vi "Begin.vi"() -> (0 "error out":errorcluster)   [LabVIEW 2013]
doc: "Called before other user functions, this VI is expected to open initial I/O refnums, load in file data, and do all program initialization. Notice that the <B>error out</B> terminal is simply used for data flow. Wiring it to other structures or subVIs ensures that this VI runs first."
uses:
  <vilib>/Rock Robotics/WPI/DriverStation/WPI_DriverStationRobotMode2.ctl
  <vilib>/Rock Robotics/WPI/Joystick/WPI_JoystickDeviceEnum.ctl
  <vilib>/Rock Robotics/SystemInterfaces/AI/FPGA_AIGyroChannel.ctl
  <vilib>/Rock Robotics/SystemInterfaces/Typedef/FPGA_TypedefAnalogModuleForGyro.ctl
  <vilib>/Rock Robotics/SystemInterfaces/DIO/FPGA_DIOChannel.ctl
  <vilib>/Rock Robotics/SystemInterfaces/DIO/FPGA_DIORelayChannel.ctl
  <vilib>/Rock Robotics/SystemInterfaces/AI/FPGA_AIChannel.ctl
  <vilib>/Rock Robotics/SystemInterfaces/DIO/FPGA_DIOPWMChannel.ctl
  <vilib>/Rock Robotics/SystemInterfaces/Typedef/FPGA_TypedefDigitalModule.ctl
  Drivetrain/Arcade Drive Ref.ctl
  <vilib>/Rock Robotics/WPI/MotorControl/WPI_MotorControlDeviceRef.ctl
  <vilib>/Rock Robotics/WPI/PWM/WPI_PWMDeadband.ctl
  <vilib>/Rock Robotics/WPI/CAN/Jaguar/SubVIs/WPI_CANJaguar_ControlMode.ctl
  <vilib>/Rock Robotics/WPI/PWM/WPI_PWMTransform_ConPane.ctl
  <vilib>/Rock Robotics/WPI/Solenoid/WPI_SolenoidChannel.ctl
  Robot Global Data.vi
  <vilib>/Rock Robotics/WPI/MotorControl/WPI_MotorControlOpen Talon.vi
  <vilib>/Rock Robotics/WPI/Counter/WPI_CounterDigitalInputToDigitalSource.vi
  <vilib>/Rock Robotics/WPI/Solenoid/WPI_SolenoidOpenSingle.vi
  <vilib>/Rock Robotics/WPI/Compressor/WPI_CompressorGetSetRefNum.vi
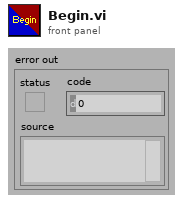
[diagram p1: front panel]
types:
  T1 = typedef "WPI_SolenoidChannel.ctl" = enum8{"Solenoid 1", "Solenoid 2", "Solenoid 3", "Solenoid 4", "Solenoid 5", "Solenoid 6", "Solenoid 7", "Solenoid 8", "Invalid"}
  T2 = typedef "Arcade Drive Ref.ctl" = cluster{"L1":T3, "L2":T3, "R1":T3, "R2":T3, "Motor Count":enum16{"2 Motor", "4 Motor"}, "L Reversed?":bool, "R Reversed?":bool}
  T3 = typedef "WPI_MotorControlDeviceRef.ctl" = cluster{"DeviceStatus":errorcluster, "Type":enum16{"PWM", "CAN"}, "PWM":cluster{"Digital Module":T4, "PWM Channel":T5, "DeadBand":T6}, "CAN":cluster{"Device Number":u8, "Control Mode":T7, "Semaphore":T8, "Max Vout":dbl}, "Invert":bool, "TransformRef":T9, "InvTransformRef":T9}
  T4 = typedef "FPGA_TypedefDigitalModule.ctl" = enum16{"Digital Module 1", "Digital Module 2"}
  T5 = typedef "FPGA_DIOPWMChannel.ctl" = enum8{"PWM 1", "PWM 2", "PWM 3", "PWM 4", "PWM 5", "PWM 6", "PWM 7", "PWM 8", "PWM 9", "PWM 10", "Invalid"}
  T6 = typedef "WPI_PWMDeadband.ctl" = cluster{"Name":string, "maxPositivePwm":i32, "minPositivePwm":i32, "centerPwm":i32, "maxNegativePwm":i32, "minNegativePwm":i32, "angularRange":u16}
  T7 = typedef "WPI_CANJaguar_ControlMode.ctl" = enum8{"Percent VBus", "Current", "Speed", "Position", "Voltage"}
  T8 = typedef "Semaphore RefNum" = refnum<k1>
  T9 = typedef "WPI_PWMTransform_ConPane.ctl" = refnum<vi>
  T10 = typedef "FPGA_DIOChannel.ctl" = enum8{"DIO 1", "DIO 2", "DIO 3", "DIO 4", "DIO 5", "DIO 6", "DIO 7", "DIO 8", "DIO 9", "DIO 10", "DIO 11", "DIO 12", "DIO 13", "DIO 14", "Invalid"}
  T11 = typedef "FPGA_AIChannel.ctl" = enum8{"AI 1", "AI 2", "AI 3", "AI 4", "AI 5", "AI 6", "AI 7", "AI 8", "Invalid"}
  T12 = typedef "FPGA_DIORelayChannel.ctl" = enum8{"Relay 1", "Relay 2", "Relay 3", "Relay 4", "Relay 5", "Relay 6", "Relay 7", "Relay 8", "Invalid"}
  T13 = typedef "WPI_JoystickDeviceEnum.ctl" = enum16{"USB 1", "USB 2", "USB 3", "USB 4", "Kinect 1", "Kinect 2"}
  T14 = typedef "FPGA_TypedefAnalogModuleForGyro.ctl" = enum16{"Analog Module 1"}
  T15 = typedef "FPGA_AIGyroChannel.ctl" = enum8{"AI 1", "AI 2", "Invalid"}
  T16 = typedef "WPI_DriverStationRobotMode2.ctl" = enum16{"Autonomous Disabled", "Autonomous Enabled", "Teleop Disabled", "Teleop Enabled", "Timeout", "Finish", "Test Disabled", "Test Enabled"}
  T17 = typedef "WPI_DigitalInputDevRef.ctl" = cluster{"DevStatus":errorcluster, "DIO Channel":T10, "Digital Module":T4}
  T18 = typedef "FPGA_CounterEncoderSourceConvertionLVSourceType.ctl" = cluster{"DevStatus":errorcluster, "AnalogTriggerMode?":bool, "DigitalMode":cluster{"Digital Module":T4, "DIO Channel":T19}, "AnalogTriggerMode":cluster{"AnalogTriggerIndex":T20, "OutputType":T21}}
  T19 = typedef "FPGA_DIODigitalSourceChannel.ctl" = enum8{"DIO 1", "DIO 2", "DIO 3", "DIO 4", "DIO 5", "DIO 6", "DIO 7", "DIO 8", "DIO 9", "DIO 10", "DIO 11", "DIO 12", "DIO 13", "DIO 14", "Disabled"}
  T20 = typedef "FPGA_AnalogTriggerIndex.ctl" = enum8{"Trig 0", "Trig 1", "Trig 2", "Trig 3", "Trig 4", "Trig 5", "Trig 6", "Trig 7", "Invalid"}
  T21 = typedef "FPGA_AnalogTriggerOutType.ctl" = enum16{"InWindow", "TriggerState", "Rising", "Falling"}
  T22 = typedef "WPI_EncoderDevRef.ctl" = cluster{"DevStatus":errorcluster, "EncoderIndex":T23, "CounterIndex":T24, "DistancePerCount":dbl, "Decoding Type":T25}
  T23 = typedef "FPGA_EncoderIdx.ctl" = enum8{"Enc 0", "Enc 1", "Enc 2", "Enc 3", "Invalid"}
  T24 = typedef "FPGA_CounterCtrSystemIndex.ctl" = enum8{"Ctr 0", "Ctr 1", "Ctr 2", "Ctr 3", "Ctr 4", "Ctr 5", "Ctr 6", "Ctr 7", "Invalid"}
  T25 = typedef "WPI_EncoderType.ctl" = enum16{"1x", "2x", "4x"}
  T26 = typedef "WPI_AnalogChannelDevRef.ctl" = cluster{"DevStatus":errorcluster, "Analog Module":T27, "Analog Channel":T11}
  T27 = typedef "FPGA_TypedefAnalogModule.ctl" = enum16{"Analog Module 1", "Analog Module 2"}
  T28 = typedef "WPI_JoystickDevRef.ctl" = cluster{"Device":T13}
  T29 = typedef "WPI_I2CDevRef.ctl" = cluster{"DevStatus":errorcluster, "Digital Module":T4, "Device Address":u8}
  T30 = typedef "WPI_SolenoidDevRef.ctl" = cluster{"DevStatus":errorcluster, "Solenoid Module":T31, "Forward Solenoid Channel":T1, "Reverse Solenoid Channel":T1}
  T31 = typedef "FPGA_TypedefSolenoidModule.ctl" = enum16{"Solenoid Module 1", "Solenoid Module 2"}
  T32 = typedef "WPI_GyroDevRef.ctl" = cluster{"DevStatus":errorcluster, "Analog Module":T27, "Analog Channel":T11, "Offset":dbl, "Gain (VoltsPerDegree/Second)":dbl}
  T33 = typedef "WPI_CompressorDevRef.ctl" = cluster{"DevStatus":errorcluster, "DigitalInputDevRef":T17, "RelayDevRef":T34}
  T34 = typedef "WPI_RelayDevRef.ctl" = cluster{"DevStatus":errorcluster, "Relay Channel":T12, "Digital Module":T4, "Relay Direction":T35}
  T35 = typedef "WPI_RelayDirection.ctl" = enum16{"Both directions", "Forward only", "Reverse only"}
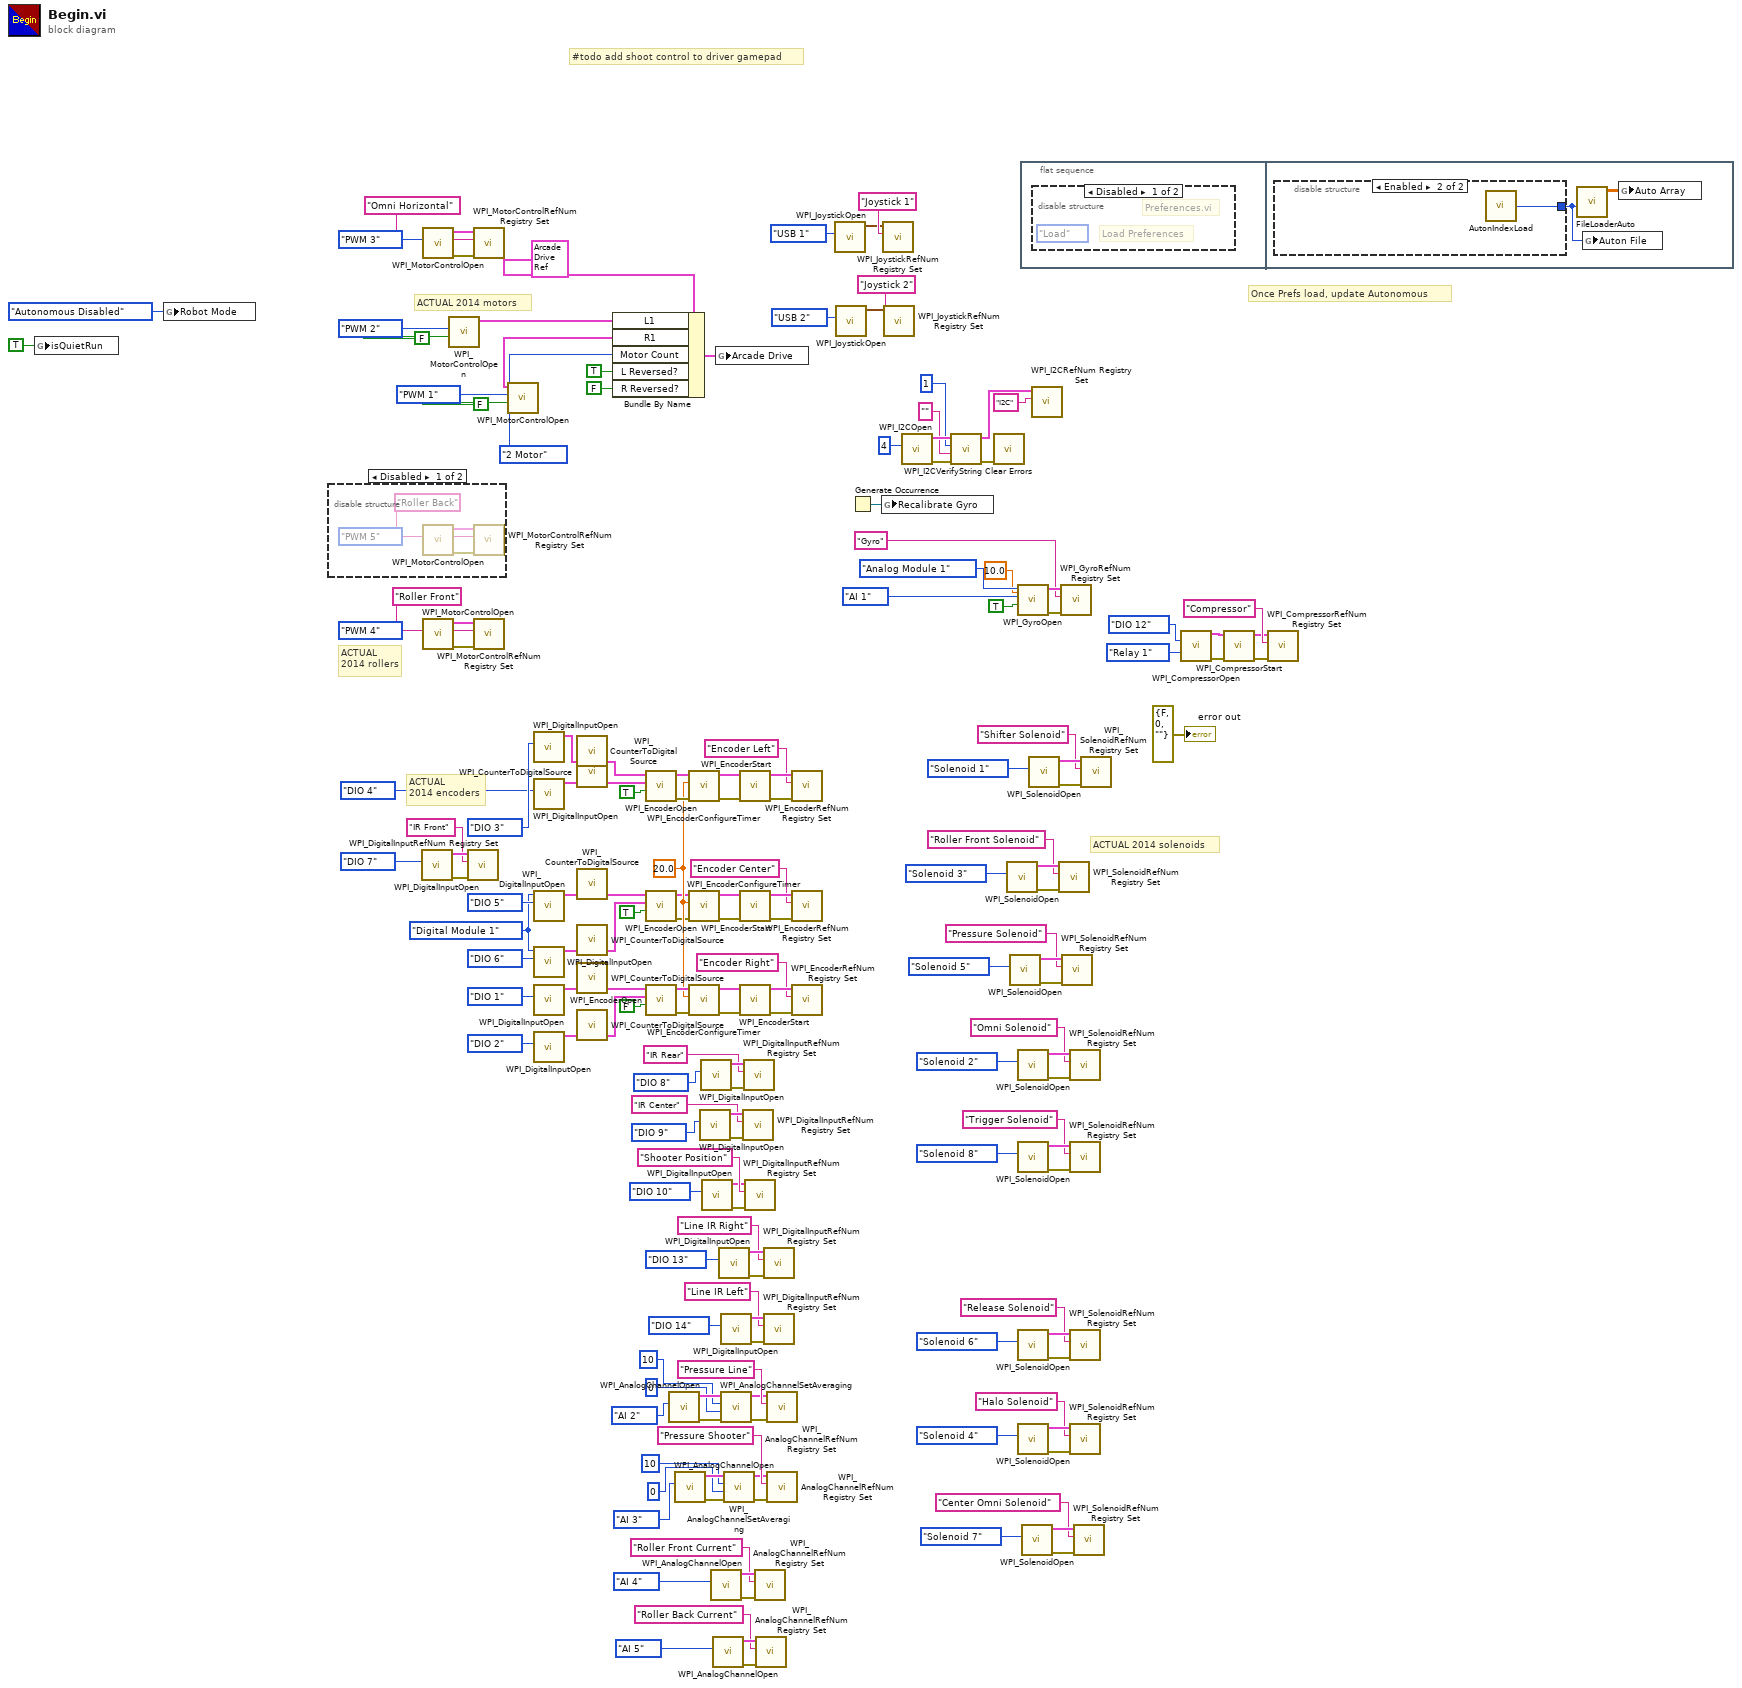
[diagram p0: block diagram]
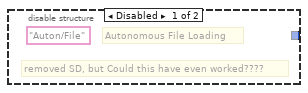
[diagram p4: hidden frame]
diagram:
  w45 = FPGA_TypedefDigitalModule."Digital Module 1" ("Digital Module (Module 1)")
  w95 = 20.0 ("Minimum Rate")
  # "ACTUAL 2014 solenoids"
  # "#todo add shoot control to driver gamepad"
  # "ACTUAL\n2014 encoders"
  # "ACTUAL\n2014 rollers"
  # "ACTUAL 2014 motors"
  # "Once Prefs load, update Autonomous"
  n1 = global write "Robot Global Data.vi" "isQuietRun"(TRUE ("isQuietRun")) -> ()
  n2 = global write "Robot Global Data.vi" "Robot Mode"(WPI_DriverStationRobotMode2."Autonomous Disabled" ("Robot Mode")) -> ()
  n3 = disable-structure shown="Disabled" {
    frame Disabled {
      n4 = call-poly <vilib>:"WPI_MotorControlOpen.vi"("PWM Channel"=FPGA_DIOPWMChannel."PWM 5") -> ("error out"=w179:errorcluster, "MotorControlDeviceRef"=w178:T3)  [unwired: 9 in]
      n5 = call <vilib>:"WPI_MotorControlRefNum Registry Set.vi"("error in (no error)"=w179, "refnum name"="Roller Back", "MotorControlDevRef"=w178) -> ()  [unwired: 7 in, 2 out]
    }
    frame Enabled {
    }
  }
  n6 = call <vilib>:"WPI_DigitalInputOpen.vi"("DIO Channel"=FPGA_DIOChannel."DIO 7") -> ("error out"=w126:errorcluster, "DigitalInputDevRef"=w125:T17)  [unwired: 9 in]
  n7 = call-poly <vilib>:"WPI_MotorControlOpen.vi"("PWM Channel"=FPGA_DIOPWMChannel."PWM 3") -> ("error out"=w49:errorcluster, "MotorControlDeviceRef"=w50:T3)  [unwired: 9 in]
  n8 = call-poly <vilib>:"WPI_MotorControlOpen.vi"("PWM Channel"=FPGA_DIOPWMChannel."PWM 4") -> ("error out"=w132:errorcluster, "MotorControlDeviceRef"=w131:T3)  [unwired: 9 in]
  n9 = call-poly <vilib>:"WPI_MotorControlOpen.vi"("Eliminate Deadband"=FALSE, "PWM Channel"=FPGA_DIOPWMChannel."PWM 2") -> ("MotorControlDeviceRef"=w53:T3)  [unwired: 8 in, 1 out]
  n10 = call <vilib>:"WPI_DigitalInputRefNum Registry Set.vi"("error in (no error)"=w126, "refnum name"="IR Front", "DigitalInputDevRef"=w125) -> ()  [unwired: 7 in, 2 out]
  n11 = call <vilib>:"WPI_MotorControlRefNum Registry Set.vi"("error in (no error)"=w49, "refnum name"="Omni Horizontal", "MotorControlDevRef"=w50) -> ()  [unwired: 7 in, 2 out]
  n12 = call <vilib>:"WPI_MotorControlRefNum Registry Set.vi"("error in (no error)"=w132, "refnum name"="Roller Front", "MotorControlDevRef"=w131) -> ()  [unwired: 7 in, 2 out]
  n13 = call-poly <vilib>:"WPI_MotorControlOpen.vi"("Eliminate Deadband"=FALSE, "PWM Channel"=FPGA_DIOPWMChannel."PWM 1") -> ("MotorControlDeviceRef"=w54:T3)  [unwired: 8 in, 1 out]
  n14 = call <vilib>:"WPI_DigitalInputOpen.vi"("DIO Channel"=FPGA_DIOChannel."DIO 3") -> ("DigitalInputDevRef"=w157:T17)  [unwired: 9 in, 1 out]
  n15 = call <vilib>:"WPI_DigitalInputOpen.vi"("DIO Channel"=FPGA_DIOChannel."DIO 4") -> ("DigitalInputDevRef"=w156:T17)  [unwired: 9 in, 1 out]
  n16 = call <vilib>:"WPI_DigitalInputOpen.vi"("DIO Channel"=FPGA_DIOChannel."DIO 5", "Digital Module (Module 1)"=w45) -> ("DigitalInputDevRef"=w46:T17)  [unwired: 8 in, 1 out]
  n17 = call <vilib>:"WPI_DigitalInputOpen.vi"("DIO Channel"=FPGA_DIOChannel."DIO 6", "Digital Module (Module 1)"=w45) -> ("DigitalInputDevRef"=w43:T17)  [unwired: 8 in, 1 out]
  n18 = call <vilib>:"WPI_DigitalInputOpen.vi"("DIO Channel"=FPGA_DIOChannel."DIO 1") -> ("DigitalInputDevRef"=w164:T17)  [unwired: 9 in, 1 out]
  n19 = call <vilib>:"WPI_DigitalInputOpen.vi"("DIO Channel"=FPGA_DIOChannel."DIO 2") -> ("DigitalInputDevRef"=w165:T17)  [unwired: 9 in, 1 out]
  n20 = call-poly <vilib>:"WPI_CounterToDigitalSource.vi"("DigitalInputDevRef"=w157) -> ("Digital Source"=w158:T18)  [unwired: 6 in]
  n21 = call-poly <vilib>:"WPI_CounterToDigitalSource.vi"("DigitalInputDevRef"=w156) -> ("Digital Source"=w155:T18)  [unwired: 6 in]
  n22 = call-poly <vilib>:"WPI_CounterToDigitalSource.vi"("DigitalInputDevRef"=w46) -> ("Digital Source"=w48:T18)  [unwired: 6 in]
  n23 = call-poly <vilib>:"WPI_CounterToDigitalSource.vi"("DigitalInputDevRef"=w43) -> ("Digital Source"=w42:T18)  [unwired: 6 in]
  n24 = call-poly <vilib>:"WPI_CounterToDigitalSource.vi"("DigitalInputDevRef"=w164) -> ("Digital Source"=w163:T18)  [unwired: 6 in]
  n25 = call-poly <vilib>:"WPI_CounterToDigitalSource.vi"("DigitalInputDevRef"=w165) -> ("Digital Source"=w166:T18)  [unwired: 6 in]
  n26 = Bundle By Name(cluster=T2 {"L1"={"DeviceStatus"={"status"=FALSE, "code"=0, "source"=""}, "Type"=enum."PWM", "PWM"={"Digital Module"=enum."Digital Module 1", "PWM Channel"=enum."PWM 1", "DeadBand"={"Name"="", "maxPositivePwm"=0, "minPositivePwm"=0, "centerPwm"=0, "maxNegativePwm"=0, "minNegativePwm"=0, "angularRange"=0}}, "CAN"={"Device Number"=0, "Control Mode"=enum."Percent VBus", "Semaphore"=refnum, "Max Vout"=0.0}, "Invert"=FALSE, "TransformRef"=refnum, "InvTransformRef"=refnum}, "L2"={"DeviceStatus"={"status"=FALSE, "code"=0, "source"=""}, "Type"=enum."PWM", "PWM"={"Digital Module"=enum."Digital Module 1", "PWM Channel"=enum."PWM 1", "DeadBand"={"Name"="", "maxPositivePwm"=0, "minPositivePwm"=0, "centerPwm"=0, "maxNegativePwm"=0, "minNegativePwm"=0, "angularRange"=0}}, "CAN"={"Device Number"=0, "Control Mode"=enum."Percent VBus", "Semaphore"=refnum, "Max Vout"=0.0}, "Invert"=FALSE, "TransformRef"=refnum, "InvTransformRef"=refnum}, "R1"={"DeviceStatus"={"status"=FALSE, "code"=0, "source"=""}, "Type"=enum."PWM", "PWM"={"Digital Module"=enum."Digital Module 1", "PWM Channel"=enum."PWM 1", "DeadBand"={"Name"="", "maxPositivePwm"=0, "minPositivePwm"=0, "centerPwm"=0, "maxNegativePwm"=0, "minNegativePwm"=0, "angularRange"=0}}, "CAN"={"Device Number"=0, "Control Mode"=enum."Percent VBus", "Semaphore"=refnum, "Max Vout"=0.0}, "Invert"=FALSE, "TransformRef"=refnum, "InvTransformRef"=refnum}, "R2"={"DeviceStatus"={"status"=FALSE, "code"=0, "source"=""}, "Type"=enum."PWM", "PWM"={"Digital Module"=enum."Digital Module 1", "PWM Channel"=enum."PWM 1", "DeadBand"={"Name"="", "maxPositivePwm"=0, "minPositivePwm"=0, "centerPwm"=0, "maxNegativePwm"=0, "minNegativePwm"=0, "angularRange"=0}}, "CAN"={"Device Number"=0, "Control Mode"=enum."Percent VBus", "Semaphore"=refnum, "Max Vout"=0.0}, "Invert"=FALSE, "TransformRef"=refnum, "InvTransformRef"=refnum}, "Motor Count"=enum."2 Motor", "L Reversed?"=FALSE, "R Reversed?"=FALSE} ("Arcade Drive"), "L1"=w53, "R1"=w54, "Motor Count"=enum16{"2 Motor", "4 Motor", ""}."2 Motor", "L Reversed?"=TRUE, "R Reversed?"=FALSE) -> (w73:T2)
  n27 = call <vilib>:"WPI_EncoderOpen.vi"("Invert Direction (False)"=TRUE, "BSource"=w155, "ASource"=w158) -> ("error out"=w160:errorcluster, "EncoderDevRef"=w159:T22)  [unwired: 7 in]
  n28 = call <vilib>:"WPI_EncoderOpen.vi"("Invert Direction (False)"=TRUE, "BSource"=w42, "ASource"=w48) -> ("error out"=w40:errorcluster, "EncoderDevRef"=w41:T22)  [unwired: 7 in]
  n29 = call <vilib>:"WPI_EncoderOpen.vi"("Invert Direction (False)"=FALSE, "BSource"=w166, "ASource"=w163) -> ("error out"=w168:errorcluster, "EncoderDevRef"=w167:T22)  [unwired: 7 in]
  n30 = call <vilib>:"WPI_AnalogChannelOpen.vi"("Analog Channel"=FPGA_AIChannel."AI 2") -> ("error out"=w84:errorcluster, "AIDeviceRef"=w83:T26)  [unwired: 9 in]
  n31 = call <vilib>:"WPI_AnalogChannelOpen.vi"("Analog Channel"=FPGA_AIChannel."AI 3") -> ("error out"=w79:errorcluster, "AIDeviceRef"=w78:T26)  [unwired: 9 in]
  n32 = call <vilib>:"WPI_EncoderConfigureTimer.vi"("error in (no error)"=w160, "Minimum Rate"=w95, "EncoderDevRef"=w159) -> ("error out"=w162:errorcluster, "EncoderDevRef"=w161:T22)  [unwired: 7 in]
  n33 = call <vilib>:"WPI_EncoderConfigureTimer.vi"("error in (no error)"=w40, "Minimum Rate"=w95, "EncoderDevRef"=w41) -> ("error out"=w38:errorcluster, "EncoderDevRef"=w39:T22)  [unwired: 7 in]
  n34 = call <vilib>:"WPI_EncoderConfigureTimer.vi"("error in (no error)"=w168, "Minimum Rate"=w95, "EncoderDevRef"=w167) -> ("error out"=w170:errorcluster, "EncoderDevRef"=w169:T22)  [unwired: 7 in]
  n35 = call <vilib>:"WPI_DigitalInputOpen.vi"("DIO Channel"=FPGA_DIOChannel."DIO 9") -> ("error out"=w130:errorcluster, "DigitalInputDevRef"=w129:T17)  [unwired: 9 in]
  n36 = call <vilib>:"WPI_DigitalInputOpen.vi"("DIO Channel"=FPGA_DIOChannel."DIO 8") -> ("error out"=w122:errorcluster, "DigitalInputDevRef"=w121:T17)  [unwired: 9 in]
  n37 = call <vilib>:"WPI_DigitalInputOpen.vi"("DIO Channel"=FPGA_DIOChannel."DIO 10") -> ("error out"=w105:errorcluster, "DigitalInputDevRef"=w104:T17)  [unwired: 9 in]
  n38 = call <vilib>:"WPI_AnalogChannelOpen.vi"("Analog Channel"=FPGA_AIChannel."AI 4") -> ("error out"=w110:errorcluster, "AIDeviceRef"=w109:T26)  [unwired: 9 in]
  n39 = call <vilib>:"WPI_AnalogChannelOpen.vi"("Analog Channel"=FPGA_AIChannel."AI 5") -> ("error out"=w114:errorcluster, "AIDeviceRef"=w113:T26)  [unwired: 9 in]
  n40 = global write "Robot Global Data.vi" "Arcade Drive"(w73) -> ()
  n41 = call <vilib>:"WPI_DigitalInputOpen.vi"("DIO Channel"=FPGA_DIOChannel."DIO 13") -> ("error out"=w94:errorcluster, "DigitalInputDevRef"=w93:T17)  [unwired: 9 in]
  n42 = call <vilib>:"WPI_DigitalInputOpen.vi"("DIO Channel"=FPGA_DIOChannel."DIO 14") -> ("error out"=w90:errorcluster, "DigitalInputDevRef"=w89:T17)  [unwired: 9 in]
  n43 = call <vilib>:"WPI_AnalogChannelSetAveraging.vi"("error in (no error)"=w84, "OversampleBits"=u8 0, "AverageBits"=u8 10, "AIDeviceRef"=w83) -> ("error out"=w86:errorcluster, "AIDeviceRef"=w85:T26)  [unwired: 6 in]
  n44 = call <vilib>:"WPI_AnalogChannelSetAveraging.vi"("error in (no error)"=w79, "OversampleBits"=u8 0, "AverageBits"=u8 10, "AIDeviceRef"=w78) -> ("error out"=w81:errorcluster, "AIDeviceRef"=w80:T26)  [unwired: 6 in]
  n45 = call <vilib>:"WPI_EncoderStart.vi"("error in (no error)"=w162, "EncoderDevRef"=w161) -> ("error out"=w154:errorcluster, "EncoderDevRef"=w153:T22)  [unwired: 8 in]
  n46 = call <vilib>:"WPI_EncoderStart.vi"("error in (no error)"=w38, "EncoderDevRef"=w39) -> ("error out"=w37:errorcluster, "EncoderDevRef"=w36:T22)  [unwired: 8 in]
  n47 = call <vilib>:"WPI_EncoderStart.vi"("error in (no error)"=w170, "EncoderDevRef"=w169) -> ("error out"=w172:errorcluster, "EncoderDevRef"=w171:T22)  [unwired: 8 in]
  n48 = call <vilib>:"WPI_DigitalInputRefNum Registry Set.vi"("error in (no error)"=w130, "refnum name"="IR Center", "DigitalInputDevRef"=w129) -> ()  [unwired: 7 in, 2 out]
  n49 = call <vilib>:"WPI_DigitalInputRefNum Registry Set.vi"("error in (no error)"=w122, "refnum name"="IR Rear", "DigitalInputDevRef"=w121) -> ()  [unwired: 7 in, 2 out]
  n50 = call <vilib>:"WPI_DigitalInputRefNum Registry Set.vi"("error in (no error)"=w105, "refnum name"="Shooter Position", "DigitalInputDevRef"=w104) -> ()  [unwired: 7 in, 2 out]
  n51 = call <vilib>:"WPI_AnalogChannelRefNum Registry Set.vi"("error in (no error)"=w110, "refnum name"="Roller Front Current", "AIDeviceRef"=w109) -> ()  [unwired: 7 in, 2 out]
  n52 = call <vilib>:"WPI_AnalogChannelRefNum Registry Set.vi"("error in (no error)"=w114, "refnum name"="Roller Back Current", "AIDeviceRef"=w113) -> ()  [unwired: 7 in, 2 out]
  n53 = call <vilib>:"WPI_DigitalInputRefNum Registry Set.vi"("error in (no error)"=w94, "refnum name"="Line IR Right", "DigitalInputDevRef"=w93) -> ()  [unwired: 7 in, 2 out]
  n54 = call <vilib>:"WPI_DigitalInputRefNum Registry Set.vi"("error in (no error)"=w90, "refnum name"="Line IR Left", "DigitalInputDevRef"=w89) -> ()  [unwired: 7 in, 2 out]
  n55 = call <vilib>:"WPI_AnalogChannelRefNum Registry Set.vi"("error in (no error)"=w86, "refnum name"="Pressure Line", "AIDeviceRef"=w85) -> ()  [unwired: 7 in, 2 out]
  n56 = call <vilib>:"WPI_AnalogChannelRefNum Registry Set.vi"("error in (no error)"=w81, "refnum name"="Pressure Shooter", "AIDeviceRef"=w80) -> ()  [unwired: 7 in, 2 out]
  n57 = call <vilib>:"WPI_EncoderRefNum Registry Set.vi"("error in (no error)"=w154, "refnum name"="Encoder Left", "EncoderDevRef"=w153) -> ()  [unwired: 7 in, 2 out]
  n58 = call <vilib>:"WPI_EncoderRefNum Registry Set.vi"("error in (no error)"=w37, "refnum name"="Encoder Center", "EncoderDevRef"=w36) -> ()  [unwired: 7 in, 2 out]
  n59 = call <vilib>:"WPI_EncoderRefNum Registry Set.vi"("error in (no error)"=w172, "refnum name"="Encoder Right", "EncoderDevRef"=w171) -> ()  [unwired: 7 in, 2 out]
  n60 = call <vilib>:"WPI_JoystickOpen.vi"("JoystickDevice"=WPI_JoystickDeviceEnum."USB 1") -> ("JoystickDevRef"=w174:T28)  [unwired: 10 in]
  n61 = call <vilib>:"WPI_JoystickOpen.vi"("JoystickDevice"=WPI_JoystickDeviceEnum."USB 2") -> ("JoystickDevRef"=w142:T28)  [unwired: 10 in]
  n62 = Generate Occurrence() -> (w74:refnum<k4>)
  n63 = global write "Robot Global Data.vi" "Recalibrate Gyro"(w74) -> ()
  n64 = call <vilib>:"WPI_JoystickRefNum Registry Set.vi"("refnum name"="Joystick 1", "JoystickDevRef"=w174) -> ()  [unwired: 8 in, 2 out]
  n65 = call <vilib>:"WPI_JoystickRefNum Registry Set.vi"("refnum name"="Joystick 2", "JoystickDevRef"=w142) -> ()  [unwired: 8 in, 2 out]
  n66 = call <vilib>:"WPI_I2COpen.vi"("Device Address"=u8 4) -> ("error out"=w69:errorcluster, "I2CDevRef"=w68:T29)  [unwired: 9 in]
  n67 = call <vilib>:"WPI_I2CVerifyString.vi"("error in (no error)"=w69, "Expected"="", "Register Address"=u8 1, "I2CDevRef"=w68) -> ("error out"=w62:errorcluster, "I2CDevRef"=w67:T29)  [unwired: 6 in]
  n68 = call <vilib>:"Clear Errors.vi"("error in (no error)"=w62) -> ()  [unwired: 6 in, 1 out]
  n69 = call-poly <vilib>:"WPI_SolenoidOpen.vi"("Solenoid Channel"=WPI_SolenoidChannel."Solenoid 3") -> ("error out"=w32:errorcluster, "SolenoidDevRef"=w31:T30)  [unwired: 9 in]
  n70 = call-poly <vilib>:"WPI_SolenoidOpen.vi"("Solenoid Channel"=WPI_SolenoidChannel."Solenoid 5") -> ("error out"=w20:errorcluster, "SolenoidDevRef"=w19:T30)  [unwired: 9 in]
  n71 = call <vilib>:"WPI_GyroOpen.vi"("Calibration Time (s)"=10.0, "Calibrate On Open"=TRUE, "Analog Channel"=FPGA_AIGyroChannel."AI 1", "Analog Module (Module 1)"=FPGA_TypedefAnalogModuleForGyro."Analog Module 1") -> ("error out"=w150:errorcluster, "GyroDevRef"=w149:T32)  [unwired: 5 in, 1 out]
  n72 = call-poly <vilib>:"WPI_SolenoidOpen.vi"("Solenoid Channel"=WPI_SolenoidChannel."Solenoid 2") -> ("error out"=w29:errorcluster, "SolenoidDevRef"=w28:T30)  [unwired: 9 in]
  n73 = call-poly <vilib>:"WPI_SolenoidOpen.vi"("Solenoid Channel"=WPI_SolenoidChannel."Solenoid 8") -> ("error out"=w12:errorcluster, "SolenoidDevRef"=w11:T30)  [unwired: 9 in]
  n74 = call-poly <vilib>:"WPI_SolenoidOpen.vi"("Solenoid Channel"=WPI_SolenoidChannel."Solenoid 6") -> ("error out"=w17:errorcluster, "SolenoidDevRef"=w16:T30)  [unwired: 9 in]
  n75 = call-poly <vilib>:"WPI_SolenoidOpen.vi"("Solenoid Channel"=WPI_SolenoidChannel."Solenoid 4") -> ("error out"=w26:errorcluster, "SolenoidDevRef"=w25:T30)  [unwired: 9 in]
  n76 = flat-sequence {
    frame #0 {
      n77 = disable-structure shown="Disabled" {
        frame Disabled {
          (unwired) enum16{"Load", "Save"}."Load" ("Operation")
          # "Preferences.vi"
          # "Load Preferences"
        }
        frame Enabled {
        }
      }
    }
    frame #1 {
      n78 = disable-structure shown="Enabled" {
        disable-tunnel: [_ w182] -> w180
        frame Disabled {
          (unwired) "Auton/File" ("Name")
          # "removed SD, but Could this have even worked????"
          # "Autonomous File Loading"
        }
        frame Enabled {
          n79 = call "AutonIndexLoad.vi"() -> ("index"=w182:i32)  [unwired: 1 in]
        }
      }
      n80 = call "FileLoaderAuto.vi"("index"=w180) -> ("Auto Array"=w181:dbl[][])  [unwired: 9 in, 1 out]
      n81 = global write "Robot Global Data.vi" "Auton File"(w180) -> ()
      n82 = global write "Robot Global Data.vi" "Auto Array"(w181) -> ()
    }
  }
  n83 = call-poly <vilib>:"WPI_SolenoidOpen.vi"("Solenoid Channel"=WPI_SolenoidChannel."Solenoid 7") -> ("error out"=w6:errorcluster, "SolenoidDevRef"=w7:T30)  [unwired: 9 in]
  n84 = call-poly <vilib>:"WPI_SolenoidOpen.vi"("Solenoid Channel"=WPI_SolenoidChannel."Solenoid 1") -> ("error out"=w4:errorcluster, "SolenoidDevRef"=w3:T30)  [unwired: 9 in]
  n85 = call <vilib>:"WPI_I2CRefNum Registry Set.vi"("refnum name"="I2C", "I2CDevRef"=w67) -> ()  [unwired: 8 in, 2 out]
  n86 = call <vilib>:"WPI_SolenoidRefNum Registry Set.vi"("error in (no error)"=w32, "refnum name"="Roller Front Solenoid", "SolenoidDevRef"=w31) -> ()  [unwired: 7 in, 2 out]
  n87 = call <vilib>:"WPI_GyroRefNum Registry Set.vi"("error in (no error)"=w150, "refnum name"="Gyro", "GyroDevRef"=w149) -> ()  [unwired: 7 in, 2 out]
  n88 = call <vilib>:"WPI_SolenoidRefNum Registry Set.vi"("error in (no error)"=w20, "refnum name"="Pressure Solenoid", "SolenoidDevRef"=w19) -> ()  [unwired: 7 in, 2 out]
  n89 = call <vilib>:"WPI_SolenoidRefNum Registry Set.vi"("error in (no error)"=w29, "refnum name"="Omni Solenoid", "SolenoidDevRef"=w28) -> ()  [unwired: 7 in, 2 out]
  n90 = call <vilib>:"WPI_SolenoidRefNum Registry Set.vi"("error in (no error)"=w12, "refnum name"="Trigger Solenoid", "SolenoidDevRef"=w11) -> ()  [unwired: 7 in, 2 out]
  n91 = call <vilib>:"WPI_SolenoidRefNum Registry Set.vi"("error in (no error)"=w17, "refnum name"="Release Solenoid", "SolenoidDevRef"=w16) -> ()  [unwired: 7 in, 2 out]
  n92 = call <vilib>:"WPI_SolenoidRefNum Registry Set.vi"("error in (no error)"=w26, "refnum name"="Halo Solenoid", "SolenoidDevRef"=w25) -> ()  [unwired: 7 in, 2 out]
  n93 = call <vilib>:"WPI_SolenoidRefNum Registry Set.vi"("error in (no error)"=w6, "refnum name"="Center Omni Solenoid", "SolenoidDevRef"=w7) -> ()  [unwired: 7 in, 2 out]
  n94 = call <vilib>:"WPI_SolenoidRefNum Registry Set.vi"("error in (no error)"=w4, "refnum name"="Shifter Solenoid", "SolenoidDevRef"=w3) -> ()  [unwired: 7 in, 2 out]
  n95 = call <vilib>:"WPI_CompressorOpen.vi"("Pressure Switch DIO Channel"=FPGA_DIOChannel."DIO 12", "Relay Channel"=FPGA_DIORelayChannel."Relay 1") -> ("CompressorDevRef"=w135:T33, "error out"=w136:errorcluster)  [unwired: 12 in]
  n96 = call <vilib>:"WPI_CompressorStart.vi"("error in (no error)"=w136, "CompressorDevRef"=w135) -> ("error out"=w133:errorcluster, "CompressorDevRef"=w134:T33)  [unwired: 8 in]
  n97 = call <vilib>:"WPI_CompressorRefNum Registry Set.vi"("error in (no error)"=w133, "refnum name"="Compressor", "CompressorDevRef"=w134) -> ()  [unwired: 7 in, 2 out]
  "error out" <- errorcluster {"status"=FALSE, "code"=0, "source"=""} ("error out")
